vi "ARC_Queue Insert Single Messenges.vi"(8 "error in (no error)":errorcluster, 9 "Data":variant, 10 "Order":string, 11 "Queue Name":string) -> (0 "error out":errorcluster)   [LabVIEW 2016]
uses:
  ARC_Queue Create_Single.vi
  ARC_Queue Insert Element.vi
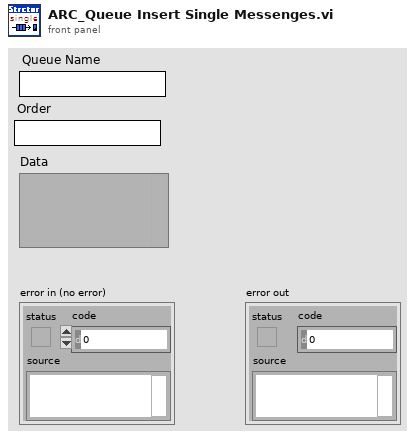
[diagram p1: front panel]
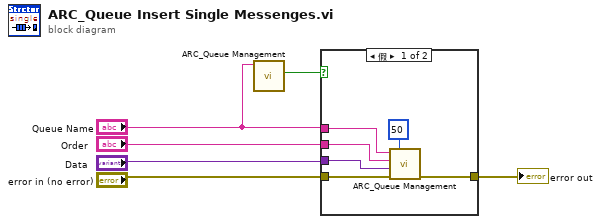
[diagram p0: block diagram]
diagram:
  n1 = call-poly "ARC_Queue Management.vi"("Queue Name"="Queue Name") -> ("Created New?"=w2:bool)  [unwired: 8 in, 2 out]
  n2 = case shown="假" w2 {
    tunnel: "error in (no error)" -> [w12 w13]
    tunnel: "Queue Name" -> [w10 _]
    tunnel: "Order" -> [w8 _]
    tunnel: "Data" -> [w9 _]
    tunnel: [w7 w13] -> w6
    frame False {
      n3 = call-poly "ARC_Queue Management.vi"("Time out(-1)_queue in"=50, "error in (no error)"=w12, "Data"=w9, "Event"=w8, "Queue Name(unamed)"=w10) -> ("error out"=w7:errorcluster)  [unwired: 5 in, 1 out]
    }
    frame True {
    }
  }
  "error out" <- w6
